vi "Next ramp and field.vi"(2 "Magnet Constants in":T1={"Switch resistant [K]"=5.0, "Switch superconducting [K]"=4.0, "First stage critical temperature [K]"=50.0, "Second stage critical temperature [K]"=5.0, "Inner magnet critical temperature [K]"=6.0, "Outer magnet critical temperature [K]"=5.0, "Field Constant [T/A]"=0.14911, "Maximum Current [A]"=107.3, "Maximum field [T]"=16.0, "Maximum source ramp [A/s]"=0.5, "Source precision [T]"=2e-05, "Ramp limits [A/s]"=[0.0506, 0.038, 0.0285, 0.0213, 0.0104], "Field limits [T]"=[3.0, 9.6, 13.3, 15.5, 16.0], "SMS"="COM3", "LSC218"="COM1"}, 4 "Actual field [T]":dbl, 5 "Desired":T2={"Field [T]"=0.0, "Ramp [T/s]"=0.0, "Custom Ramp?"=TRUE, "Mode"=enum."Persistant"}) -> (0 "Ramp to set [A/s]":dbl, 1 "Field to set [T]":dbl)   [LabVIEW 2021, in "Magnet module.lvlib"]
doc: "Evaluates what should be a next field target and ramp, to achoved desired value."
uses:
  Magnet module.lvlib
  ctl/SetField data.ctl
  ctl/Magnet mode public.ctl
  ctl/Magnet config constants.ctl
  submodules/PSU controller/PSU controller.lvlib
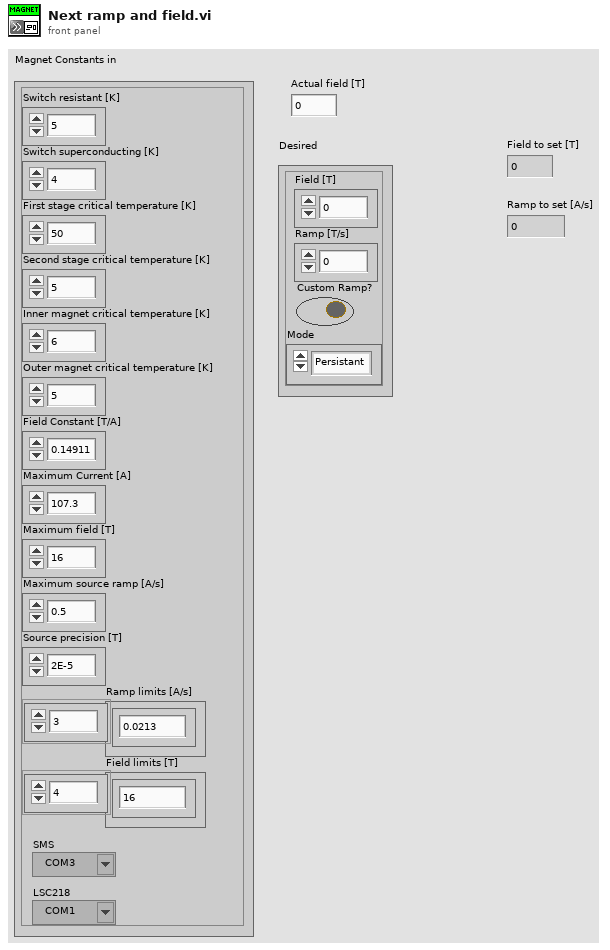
[diagram p1: front panel]
types:
  T1 = typedef "Magnet module.lvlib/Magnet config constants.ctl" = cluster{"Switch resistant [K]":dbl, "Switch superconducting [K]":dbl, "First stage critical temperature [K]":dbl, "Second stage critical temperature [K]":dbl, "Inner magnet critical temperature [K]":dbl, "Outer magnet critical temperature [K]":dbl, "Field Constant [T/A]":dbl, "Maximum Current [A]":dbl, "Maximum field [T]":dbl, "Maximum source ramp [A/s]":dbl, "Source precision [T]":dbl, "Ramp limits [A/s]":dbl[], "Field limits [T]":dbl[], "SMS":refnum<visa-resource-name>, "LSC218":refnum<visa-resource-name>}
  T2 = typedef "Magnet module.lvlib/SetField data.ctl" = cluster{"Field [T]":dbl, "Ramp [T/s]":dbl, "Custom Ramp?":bool, "Mode":T3}
  T3 = typedef "Magnet module.lvlib/Magnet mode public.ctl" = enum16{"Persistant", "Ramping"}
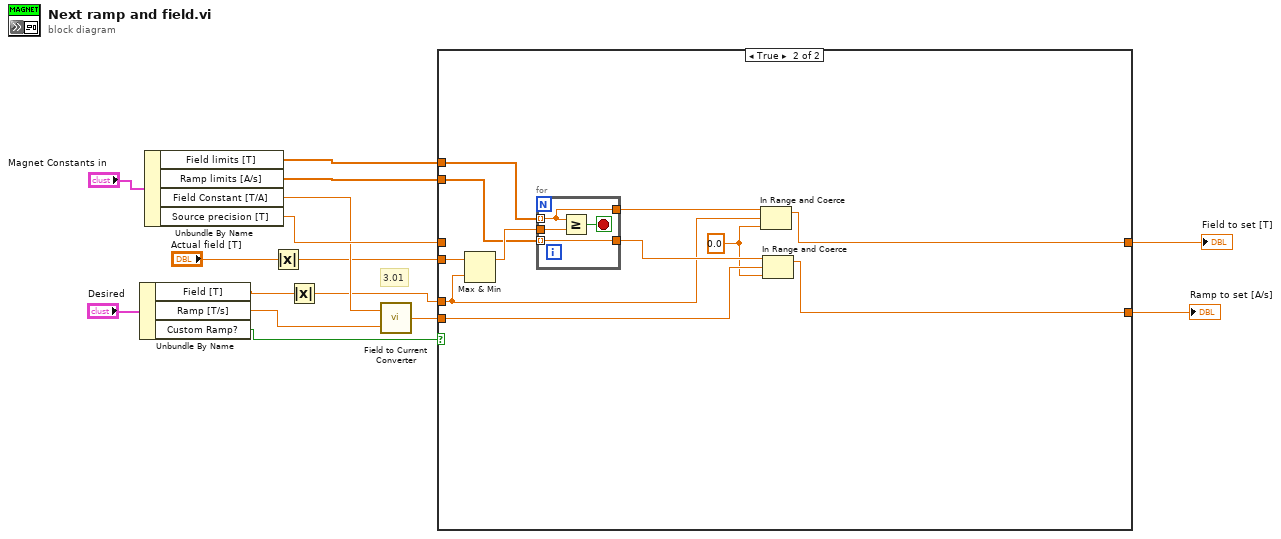
[diagram p0: block diagram]
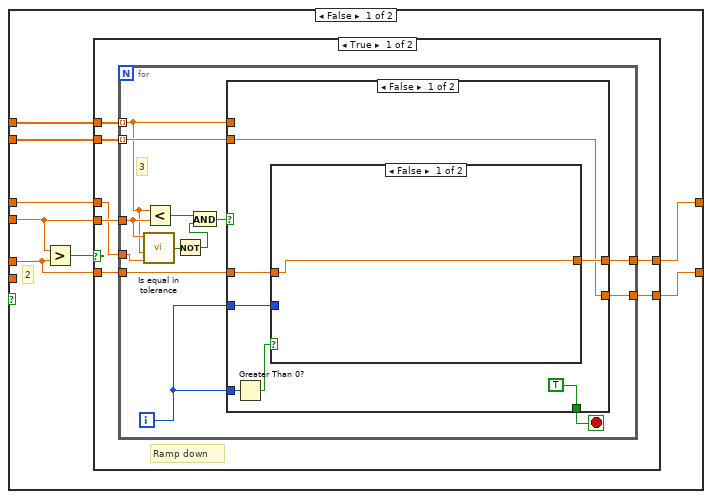
[diagram p2: hidden frame]
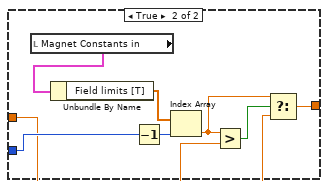
[diagram p3: hidden frame]
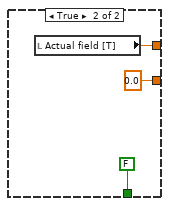
[diagram p4: hidden frame]
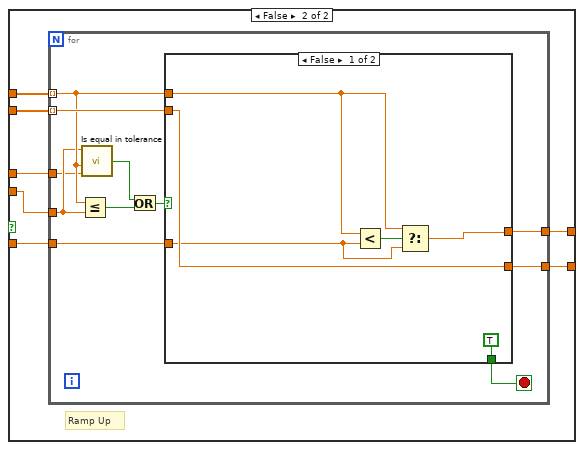
[diagram p5: hidden frame]
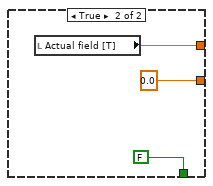
[diagram p6: hidden frame]
diagram:
  # "3.01"
  n1 = Unbundle By Name("Desired") -> ("Field [T]"=w11:dbl, "Ramp [T/s]"=w5:dbl, "Custom Ramp?"=w9:bool)
  n2 = Unbundle By Name("Magnet Constants in") -> ("Field limits [T]"=w13:dbl[], "Ramp limits [A/s]"=w12:dbl[], "Field Constant [T/A]"=w3:dbl, "Source precision [T]"=w4:dbl)
  n3 = Absolute Value(x="Actual field [T]") -> (abs(x)=w1:dbl)
  n4 = Absolute Value(x=w11) -> (abs(x)=w2:dbl)
  n5 = call "Field to Current Converter.vi"("Field[T]"=w5, "Field constant[T/A]"=w3) -> ("Current[A]"=w6:dbl)
  n6 = case shown="True" w9 {
    tunnel: [w23 w94] -> w15
    tunnel: [w22 w93] -> w14
    tunnel: w13 -> [w21 w99]
    tunnel: w12 -> [w20 w97]
    tunnel: w2 -> [w19 w91]
    tunnel: w1 -> [w18 w100]
    tunnel: w6 -> [_ w95]
    tunnel: w4 -> [w16 _]
    frame False {
      # "2"
      n7 = Greater?(x=w18, y=w19) -> (0:w17:bool)
      n8 = case shown="True" w17 {
        tunnel: w18 -> [w29 w69]
        tunnel: w20 -> [w28 w68]
        tunnel: w21 -> [w30 w66]
        tunnel: [w27 w67] -> w23
        tunnel: w19 -> [w25 w64]
        tunnel: [w26 w65] -> w22
        tunnel: w16 -> [w24 w63]
        frame True {
          # "Ramp down"
          n9 = for {
            tunnel: w30 -> [w36] mode=indexing
            tunnel: w29 -> [w37]
            tunnel: w28 -> [w39] mode=indexing
            tunnel: [w43] -> w27
            tunnel: [w41] -> w26
            tunnel: w25 -> [w38]
            tunnel: w24 -> [w35]
            i -> [w40]
            stop <- w42 stop-if-true
            # "3"
            n10 = call "Is equal in tolerance.vi"("Absolut tolerance"=w35, "Reference value"=w36, "Input value"=w37) -> ("Is in range"=w34:bool)  [unwired: 1 in]
            n11 = Less?(x=w36, y=w37) -> (x < y?=w32:bool)
            n12 = Not(x=w34) -> (.not. x?=w33:bool)
            n13 = And(x=w32, y=w33) -> (x .and. y?=w31:bool)
            n14 = case shown="False" w31 {
              tunnel: w36 -> [_ _]
              tunnel: [w45 0.0 ("Numeric")] -> w43
              tunnel: [TRUE FALSE] -> w42
              tunnel: [w47 w60] -> w41
              tunnel: w40 -> [w50 _]
              tunnel: w40 -> [w48 _]
              tunnel: w39 -> [w45 _]
              tunnel: w38 -> [w44 _]
              frame False {
                n15 = Greater Than 0?(x=w50) -> (x > 0?=w49:bool)
                n16 = case shown="False" w49 {
                  tunnel: w48 -> [_ w59]
                  tunnel: [w51 w57] -> w47
                  tunnel: w44 -> [w51 w52]
                  frame False {
                  }
                  frame True {
                    n17 = local read "Magnet Constants in"() -> (w56:T1)
                    n18 = Unbundle By Name(w56) -> ("Field limits [T]"=w55:dbl[])
                    n19 = Decrement(x=w59) -> (x-1=w58:i32)
                    n20 = Index Array(array=w55, index=w58) -> (element=w54:dbl)
                    n21 = Greater?(x=w54, y=w52) -> (0:w53:bool)
                    n22 = Select(t=w54, s=w53, f=w52) -> (s? t:f=w57:dbl)
                  }
                }
              }
              frame True {
                n23 = local read "Actual field [T]"() -> (w60:dbl)
              }
            }
          }
        }
        frame False {
          # "Ramp Up"
          n24 = for {
            tunnel: w69 -> [w74]
            tunnel: w68 -> [w77] mode=indexing
            tunnel: [w80] -> w67
            tunnel: w66 -> [w75] mode=indexing
            tunnel: [w78] -> w65
            tunnel: w64 -> [w76]
            tunnel: w63 -> [w73]
            stop <- w79 stop-if-true
            n25 = Less Or Equal?(x=w75, y=w74) -> (x <= y?=w71:bool)
            n26 = call "Is equal in tolerance.vi"("Absolut tolerance"=w73, "Reference value"=w75, "Input value"=w74) -> ("Is in range"=w70:bool)  [unwired: 1 in]
            n27 = Or(x=w70, y=w71) -> (x .or. y?=w72:bool)
            n28 = case shown="False" w72 {
              tunnel: w75 -> [w82 _]
              tunnel: [w84 0.0 ("Numeric")] -> w80
              tunnel: [TRUE FALSE] -> w79
              tunnel: w77 -> [w84 _]
              tunnel: [w85 w87] -> w78
              tunnel: w76 -> [w81 _]
              frame False {
                n29 = Less?(x=w82, y=w81) -> (x < y?=w83:bool)
                n30 = Select(t=w82, s=w83, f=w81) -> (s? t:f=w85:dbl)
              }
              frame True {
                n31 = local read "Actual field [T]"() -> (w87:dbl)
              }
            }
          }
        }
      }
    }
    frame True {
      w90 = 0.0 ("lower limit")
      n32 = Max & Min(x=w100, y=w91) -> (max(x,y)=w98:dbl)  [unwired: 1 out]
      n33 = for {
        tunnel: w99 -> [w103] mode=indexing
        tunnel: w98 -> [w102]
        tunnel: w97 -> [w104] mode=indexing
        tunnel: [w104] -> w96
        tunnel: [w103] -> w92
        stop <- w101 stop-if-true
        n34 = Greater Or Equal?(x=w103, y=w102) -> (x >= y?=w101:bool)
      }
      n35 = In Range and Coerce(upper limit=w92, x=w91, lower limit=w90) -> (coerced(x)=w93:dbl)  [unwired: 1 out]
      n36 = In Range and Coerce(upper limit=w96, x=w95, lower limit=w90) -> (coerced(x)=w94:dbl)  [unwired: 1 out]
    }
  }
  "Ramp to set [A/s]" <- w15
  "Field to set [T]" <- w14
